vi "Ver 1.2.vi"() -> ()   [LabVIEW 2015]
uses:
  <instrlib>/Keithley 622x LV 2009/Configure/Source/Typedefs/KE622x -- Voltage Limit.ctl
  <instrlib>/Keithley 622x LV 2009/Configure/Source/Typedefs/KE622x -- Current Range.ctl
  <instrlib>/Keithley 622x LV 2009/Configure/Source/Typedefs/KE622x -- Current Ranges.ctl
  <instrlib>/Keithley 622x LV 2009/Typedefs/KE622x -- On Off Control.ctl
  <instrlib>/Keithley 622x LV 2009/Utility/Typedefs/KE622x -- Instrument Type.ctl
  <instrlib>/Keithley 622x LV 2009/Configure/Source/Typedefs/KE622x -- Current Level.ctl
  <instrlib>/Keithley 2000/Public/Configure/Configure DC Volts.vi
  <instrlib>/Keithley 2000/Keithley 2000.lvlib
  <instrlib>/Keithley 622x LV 2009/Keithley 622x.lvlib
panel:
  out "LIMIT":bool
  out "LIMIT":bool
  out "Error Code":string
  in  "Comments":string
  out "file":refnum<file>
  in  "Custom Range (0 V) 2":dbl format="%#_6p"
  in  "Auto\nRange 2":bool
  out "2000":refnum<visa-resource-name>
  out "6221":refnum<visa-resource-name>
  in  "Floating-point file recording":bool
  in  "Step  (A)":dbl=5e-05 format="%#_3p"
  in  "Stop\ncurrent (A)":dbl=0.002 format="%#_6p"
  in  "Start \ncurrent (A)":dbl=0.001 format="%#_6p"
  out "?":string
  out "?":string
  in  "Change Volt Ampers":bool
  in  "Check For SCPI Errors? (T)":bool=TRUE
  out "Interlock Tripped?":bool
  out "Compliance?":bool
  in  "Turn Off Output \nIf Compliance?":bool=TRUE
  in  "Turning ON/OFF\ncurrent output":T1=enum."On"
  out "?":cluster{dbl[], dbl[]}[](graph)
  in  "Range Selection":T2={"Auto Range?"=TRUE, "Man / Selected\nRange"=enum."2nA"}
  in  "Voltage Limit (V) 3":T4=10.0 min=0.1 max=105.0 step=0.01 format="%.2p"
  in  "Interval (s)":dbl=1.0 min=1.0
  out "?":cluster{T4[], T4[]}(graph)
  # "FILE CONFIGURATION"
  # "ADMIN PANEL"
  # "KEITHLEY 6221 CONFIGURATION (ADMIN ONLY)"
  # "I don't know what the hell it is,\njust don't touch it"
  # "START, STOP, STEP, CONFIGURATION"
  # "IF ON"
  # "Compliance = Limiting output voltage\nThis switch determines if we want to switch \noff the current output if wee exceed compliance"
  # "There is a safe switch at \nthe back of the instrument \nThis indicator shows if it is on"
  # "You have hit a damn jackpot \nby exceeding the limited voltage\nCongrats"
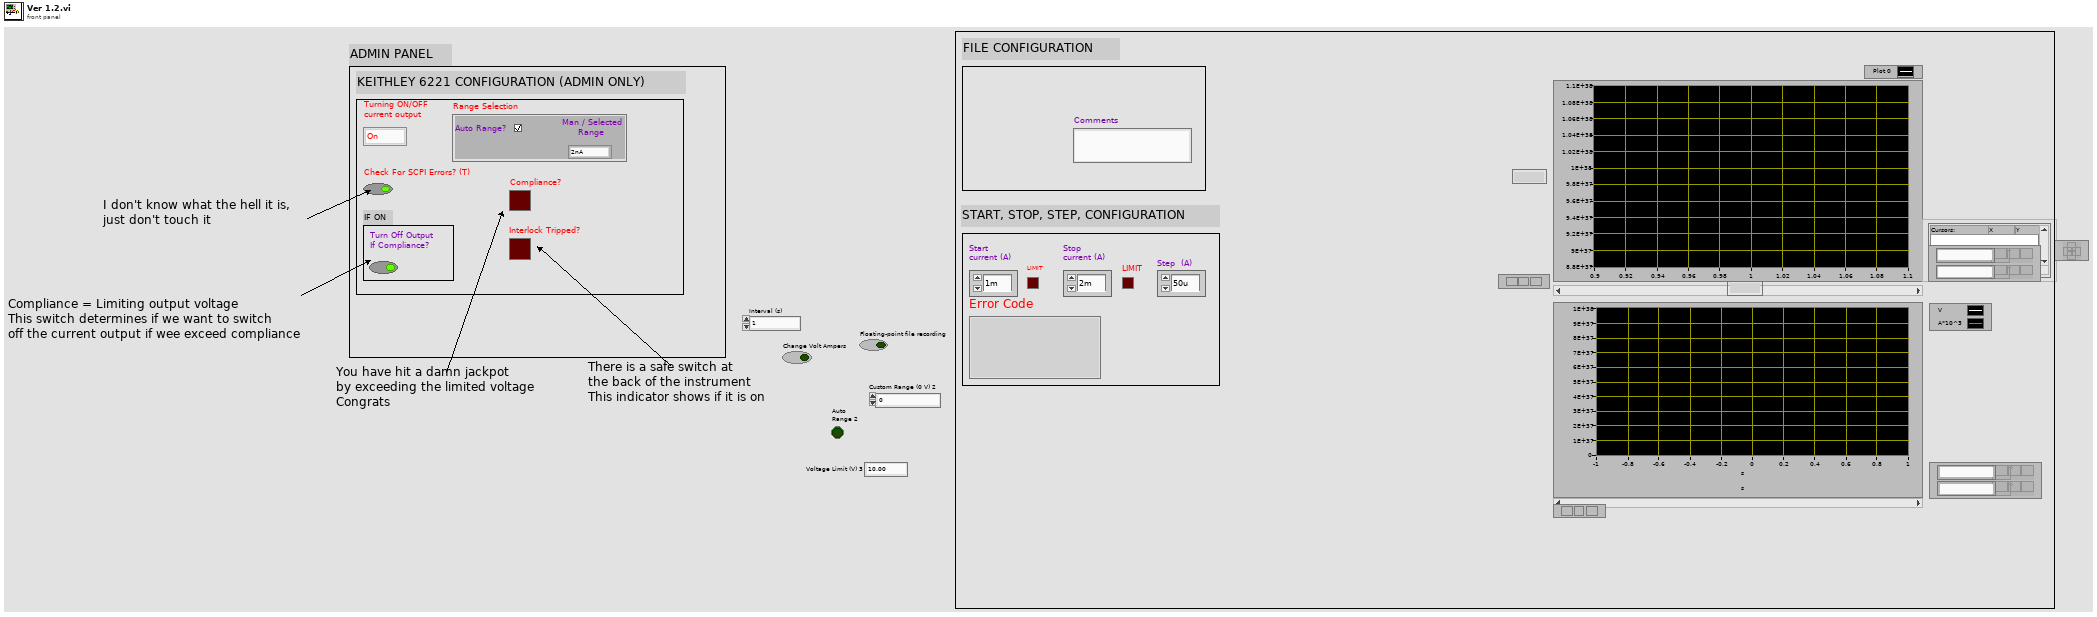
[diagram p1: front panel]
types:
  T1 = typedef "Keithley 622x.lvlib/KE622x -- On Off Control.ctl" = enum16{"Off", "On"}
  T2 = typedef "Keithley 622x.lvlib/KE622x -- Current Range.ctl" = cluster{"Auto Range?":bool, "Man / Selected\nRange":T3}
  T3 = typedef "Keithley 622x.lvlib/KE622x -- Current Ranges.ctl" = enum16{"2nA", "20nA", "200nA", "2uA", "20uA", "200uA", "2mA", "20mA", "100mA"}
  T4 = typedef "Keithley 622x.lvlib/KE622x -- Voltage Limit.ctl" = dbl
  T5 = typedef "Keithley 622x.lvlib/KE622x -- Instrument Type.ctl" = enum16{"KE6220", "KE6221"}
  T6 = typedef "Keithley 622x.lvlib/KE622x -- Current Level.ctl" = dbl
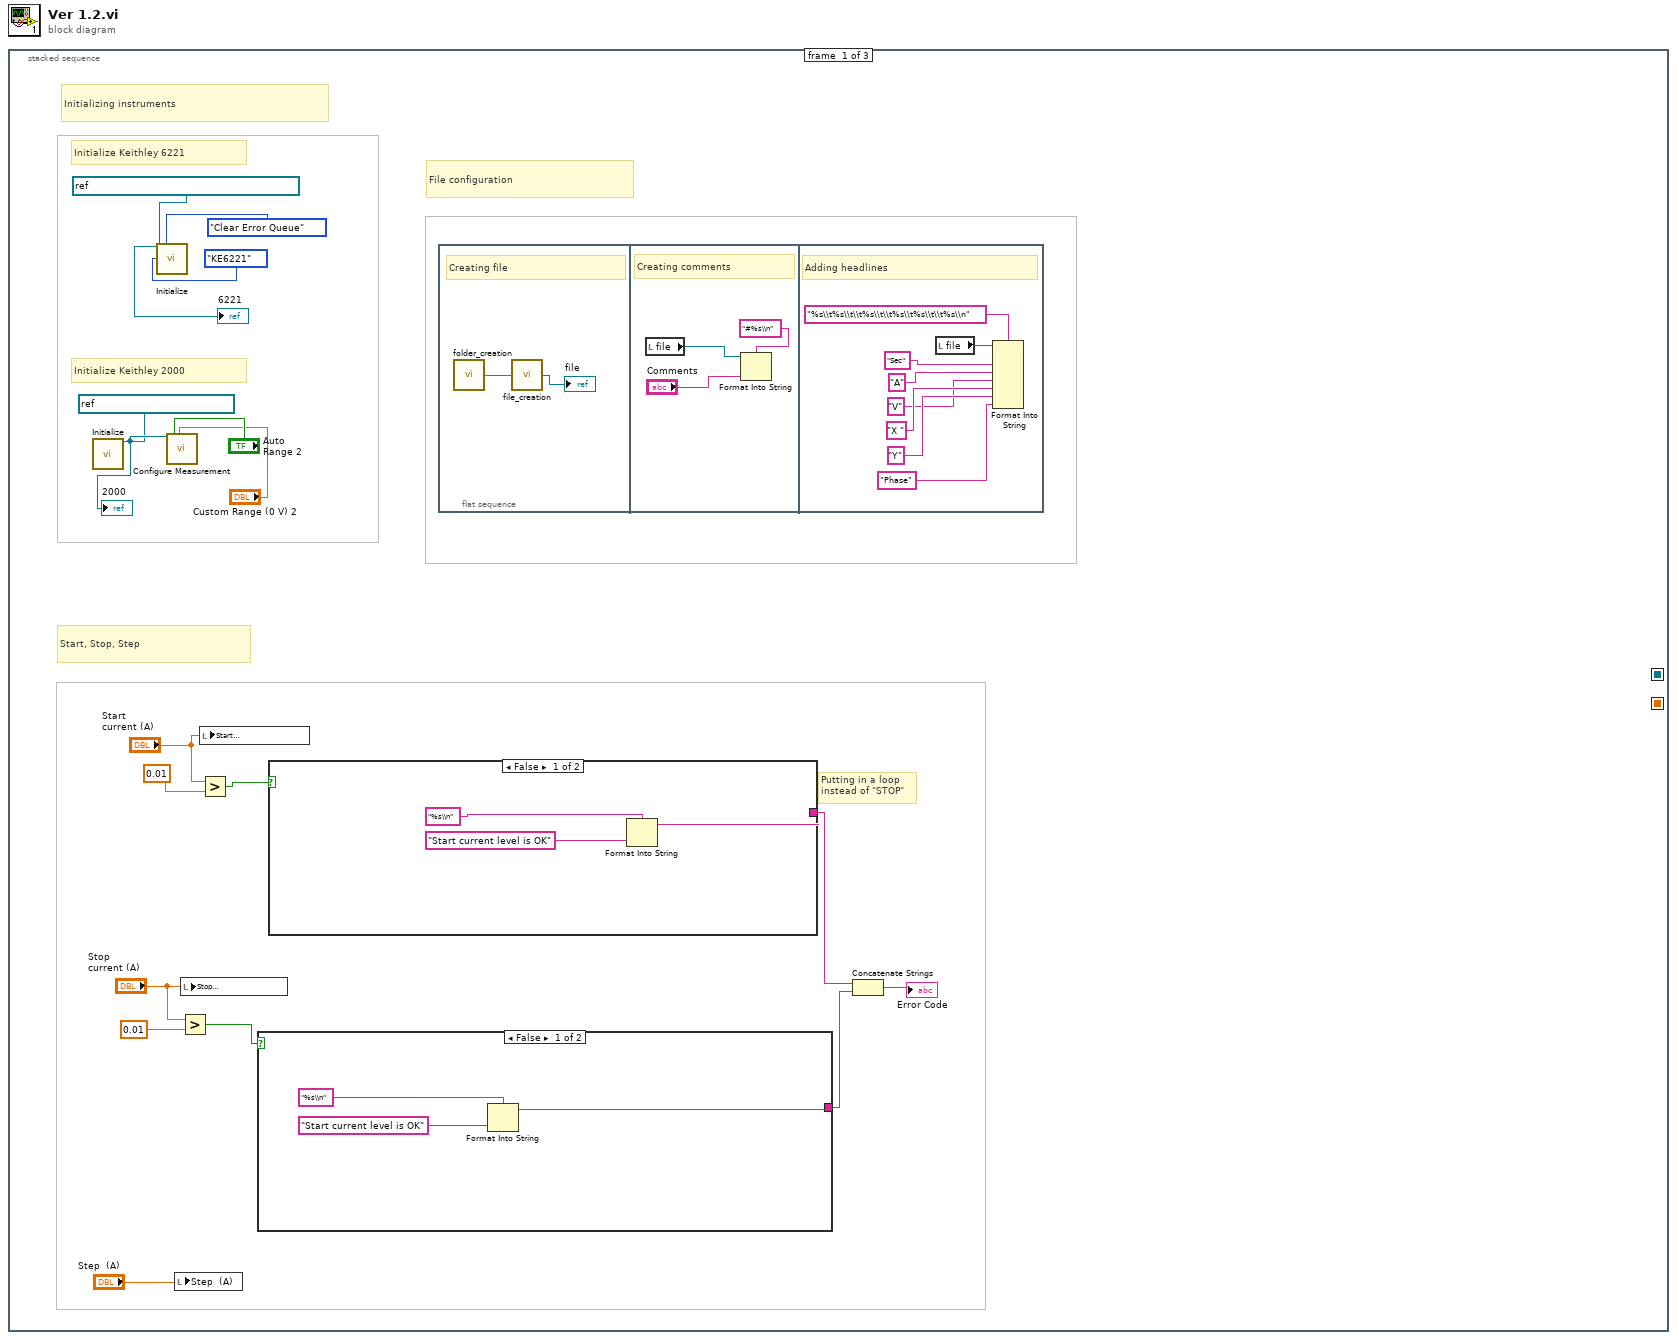
[diagram p0: block diagram]
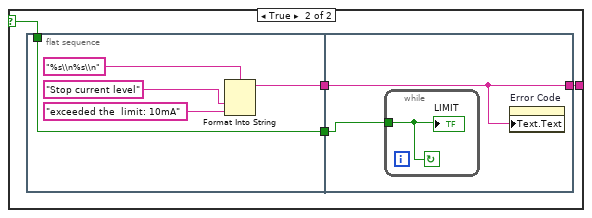
[diagram p2: hidden frame]
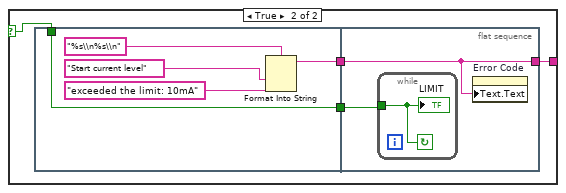
[diagram p3: hidden frame]
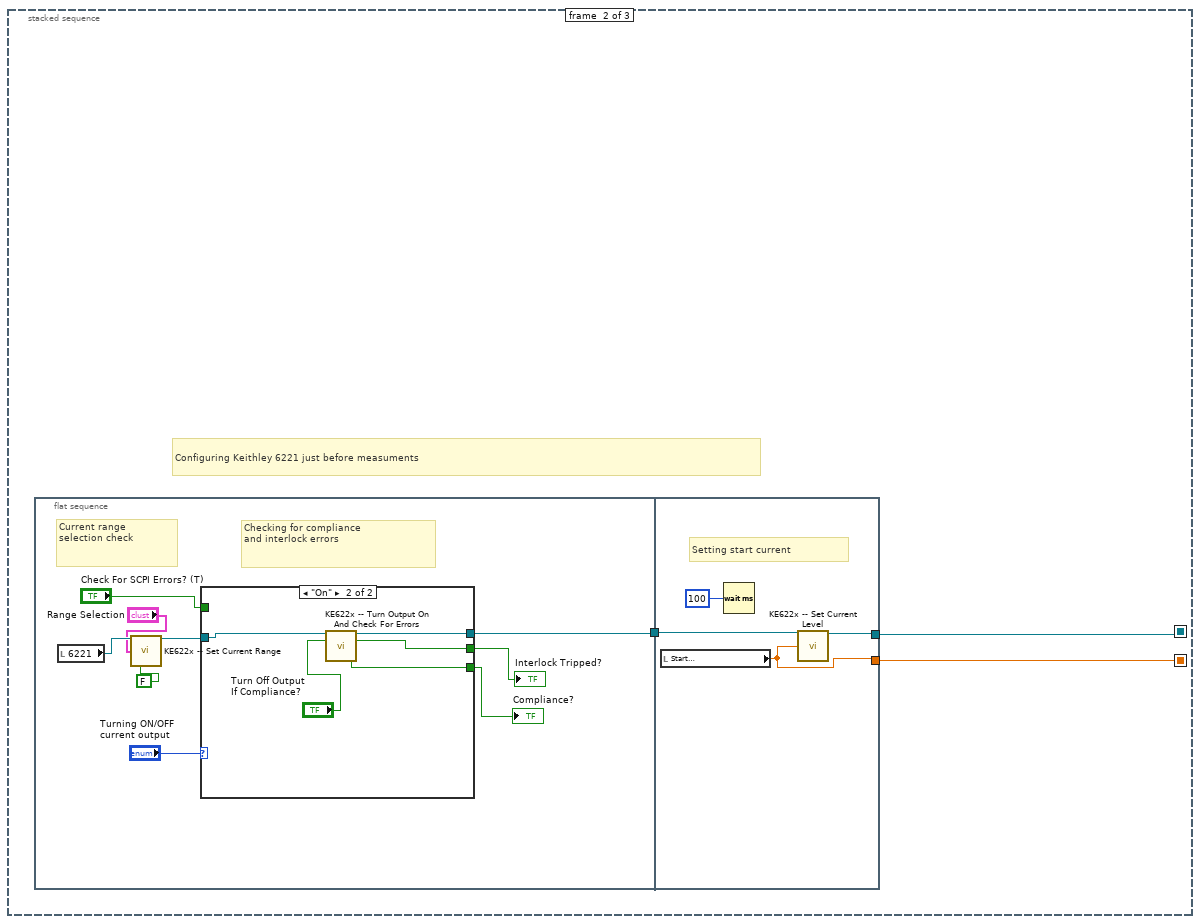
[diagram p4: hidden frame]
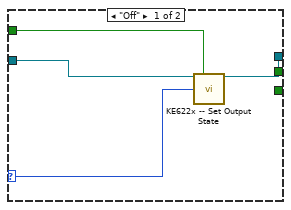
[diagram p5: hidden frame]
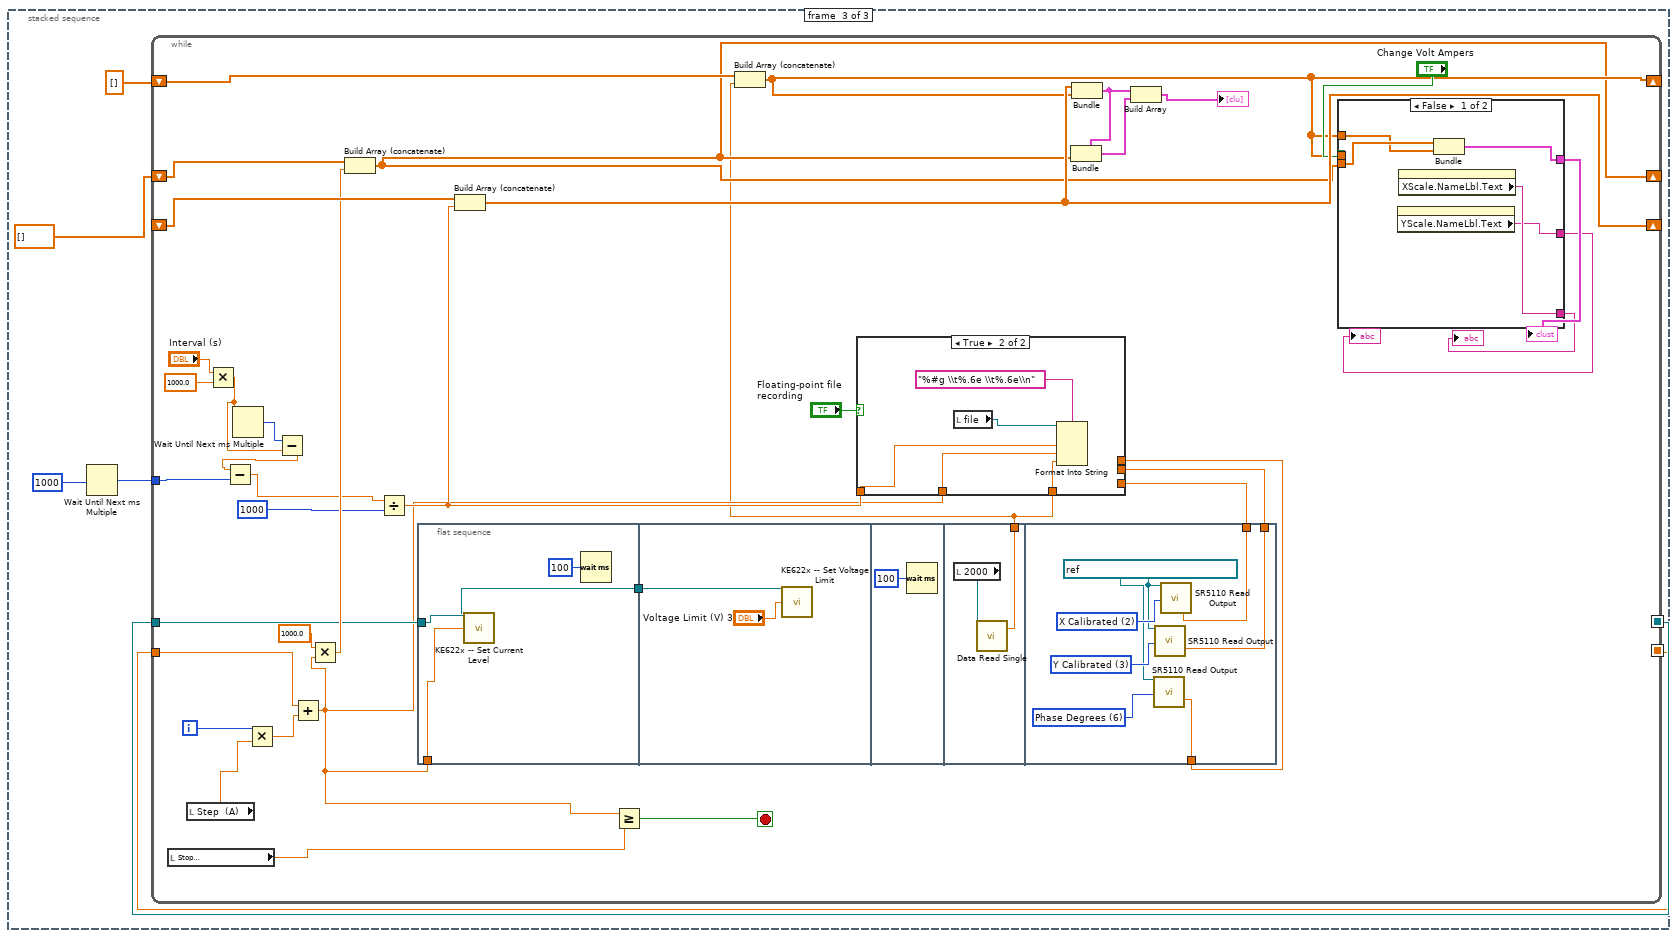
[diagram p6: hidden frame]
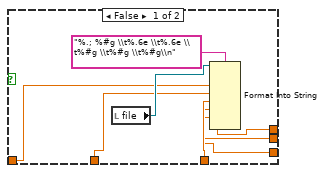
[diagram p7: hidden frame]
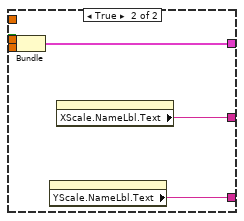
[diagram p8: hidden frame]
diagram:
  n1 = stacked-sequence {
    seq-local: [_ w64 _] -> [_ _ w87]
    seq-local: [_ w63 _] -> [_ _ w88]
    frame #0 {
      # "Putting in a loop \ninstead of \"STOP\""
      # "Start, Stop, Step"
      # "Initializing instruments"
      # "File configuration"
      # "Initialize Keithley 2000"
      # "Initialize Keithley 6221"
      n2 = call <instrlib>:"Initialize.vi"("VISA resource name"=refnum<visa-resource-name> "KEITHLEY_MULTIMETER") -> ("VISA resource name out"=w14:refnum<visa-resource-name>)  [unwired: 17 in, 1 out]
      "2000" <- w14
      n3 = call <instrlib>:"Initialize.vi"("VISA resource name"=refnum<visa-resource-name> "KEITHLEY_DC_AC_CURRENT_SOURCE", "Error Queue Option"=enum16{"Clear Error Queue", "Error Query"}."Clear Error Queue", "Instrument Type"=KE622x_--_Instrument_Type."KE6221") -> ("VISA resource name out"=→"6221":refnum<visa-resource-name>)  [unwired: 11 in, 1 out]
      n4 = call-poly <instrlib>:"Configure Measurement.vi"("VISA resource name"=w14, "Auto Range? (T: Auto)"="Auto\nRange 2", "Custom Range (0 V)"="Custom Range (0 V) 2") -> ()  [unwired: 15 in, 2 out]
      n5 = local write "Step  (A)"("Step  (A)") -> ()
      n6 = Greater?(x="Stop\ncurrent (A)", y=T4 0.01) -> (0:w4:bool)
      n7 = local write "Stop\ncurrent (A)"("Stop\ncurrent (A)") -> ()
      n8 = local write "Start \ncurrent (A)"("Start \ncurrent (A)") -> ()
      n9 = Greater?(x="Start \ncurrent (A)", y=T4 0.01) -> (0:w5:bool)
      n10 = case shown="False" w4 {
        selector: w4 -> [_ w22]
        tunnel: [w19 w25] -> w2
        frame False {
          n11 = Format Into String(format string="%s\\n", "Start current level is OK" ("false string")) -> (resulting string=w19:string)  [unwired: 2 in, 1 out]
        }
        frame True {
          n12 = flat-sequence {
            tunnel: [w27] -> w24
            tunnel: [w26] -> w23
            tunnel: w22 -> [w26]
            tunnel: [w31] -> w25
            tunnel: w24 -> [w31]
            tunnel: w23 -> [w32]
            frame #0 {
              n13 = Format Into String(format string="%s\\n%s\\n", "Stop current level" ("String"), "exceeded the  limit: 10mA" ("input 2")) -> (resulting string=w27:string)  [unwired: 2 in, 1 out]
            }
            frame #1 {
              n14 = while {
                tunnel: w32 -> [w33]
                stop <- w33 continue-if-true
                "LIMIT" <- w33
              }
              n15 = property on="Error Code" class="Str"("Text.Text"=w31) -> ()  [unwired: 2 in, 2 out]
            }
          }
        }
      }
      n16 = case shown="False" w5 {
        selector: w5 -> [_ w38]
        tunnel: [w34 w40] -> w3
        frame False {
          n17 = Format Into String(format string="%s\\n", "Start current level is OK" ("false string")) -> (resulting string=w34:string)  [unwired: 2 in, 1 out]
        }
        frame True {
          n18 = flat-sequence {
            tunnel: [w42] -> w39
            tunnel: w38 -> [w41]
            tunnel: [w41] -> w37
            tunnel: [w46] -> w40
            tunnel: w39 -> [w46]
            tunnel: w37 -> [w47]
            frame #0 {
              n19 = Format Into String(format string="%s\\n%s\\n", "Start current level" ("String"), "exceeded the limit: 10mA" ("input 2")) -> (resulting string=w42:string)  [unwired: 2 in, 1 out]
            }
            frame #1 {
              n20 = while {
                tunnel: w47 -> [w48]
                stop <- w48 continue-if-true
                "LIMIT" <- w48
              }
              n21 = property on="Error Code" class="Str"("Text.Text"=w46) -> ()  [unwired: 2 in, 2 out]
            }
          }
        }
      }
      n22 = flat-sequence {
        frame #0 {
          # "Creating file"
          n23 = call "folder_creation.vi"() -> ("String"=w50:string)
          n24 = call "file_creation.vi"("String"=w50) -> ("refnum out"=→"file":refnum<file>)
        }
        frame #1 {
          # "Creating comments"
          n25 = local read "file"() -> (w51:refnum<file>)
          n26 = Format Into String(format string="#%s\\n", initial string=w51, "Comments") -> ()  [unwired: 1 in, 2 out]
        }
        frame #2 {
          # "Adding headlines"
          n27 = local read "file"() -> (w61:refnum<file>)
          n28 = Format Into String(format string="%s\\t%s\\t\\t%s\\t\\t%s\\t%s\\t\\t%s\\n", initial string=w61, "Sec" ("input 1"), "A" ("input 2"), "V" ("input 3"), "X " ("input 3"), "Y" ("input 3"), "Phase" ("input 3")) -> ()  [unwired: 1 in, 2 out]
        }
      }
      n29 = Concatenate Strings(w3, w2) -> (→"Error Code":string)
    }
    frame #1 {
      # "Configuring Keithley 6221 just before measuments"
      n30 = flat-sequence {
        tunnel: [w65] -> w62
        tunnel: [w83] -> w64
        tunnel: [w85] -> w63
        tunnel: w62 -> [w84]
        frame #0 {
          # "Current range \nselection check"
          # "Checking for compliance\nand interlock errors"
          n31 = local read "6221"() -> (w68:refnum<visa-resource-name>)
          n32 = call <instrlib>:"KE622x -- Set Current Range.vi"("Resource In"=w68, "Current Range In"="Range Selection", "Read Back Set Values? (T)"=FALSE) -> ("Resource Out (dupl)"=w73:refnum<visa-resource-name>)  [unwired: 10 in, 2 out]
          n33 = case shown="\"On\"" "Turning ON/OFF\ncurrent output" {
            selector: "Turning ON/OFF\ncurrent output" -> [w77 _]
            tunnel: [_ w81] -> w71
            tunnel: [_ w80] -> w72
            tunnel: "Check For SCPI Errors? (T)" -> [w76 _]
            tunnel: w73 -> [w74 w79]
            tunnel: [w75 w78] -> w65
            frame "Off" {
              n34 = call <instrlib>:"KE622x -- Set Output State.vi"("Resource In"=w74, "Check For SCPI Errors? (T)"=w76, "Output State"=w77) -> ("Resource Out (dupl)"=w75:refnum<visa-resource-name>)  [unwired: 11 in, 1 out]
            }
            frame "On" {
              n35 = call <instrlib>:"KE622x -- Turn Output On And Check For Errors.vi"("Resource In"=w79, "Turn Off Output If Compliance?"="Turn Off Output \nIf Compliance?") -> ("Resource Out (dupl)"=w78:refnum<visa-resource-name>, "Interlock Tripped?"=w81:bool, "Compliance?"=w80:bool)  [unwired: 10 in, 1 out]
            }
          }
          "Interlock Tripped?" <- w71
          "Compliance?" <- w72
        }
        frame #1 {
          # "Setting start current"
          n36 = local read "Start \ncurrent (A)"() -> (w83:dbl)
          n37 = Wait (ms)(milliseconds to wait=u32 100) -> ()  [unwired: 1 out]
          n38 = call <instrlib>:"KE622x -- Set Current Level.vi"("Resource In"=w84, "Current Level (A) In"=w83) -> ("Resource Out (dupl)"=w85:refnum<visa-resource-name>)  [unwired: 12 in, 1 out]
        }
      }
    }
    frame #2 {
      n39 = Wait Until Next ms Multiple(millisecond multiple=u32 1000) -> (millisecond timer value=w89:u32)
      n40 = while {
        shift-right: [w121] -> _
        shift-left: dbl[] [] -> [w130]
        shift-right: [w126] -> _
        shift-left: _ -> [w128]
        shift-right: [w116] -> _
        shift-left: T6[] [] -> [w127]
        tunnel: w88 -> [w109]
        tunnel: w89 -> [w104]
        tunnel: w87 -> [w95]
        i -> [w118]
        stop <- w93 stop-if-true
        n41 = local read "Stop\ncurrent (A)"() -> (w94:dbl)
        n42 = local read "Step  (A)"() -> (w96:dbl)
        n43 = Multiply(x="Interval (s)", y=1000.0) -> (x*y=w105:dbl)
        n44 = Wait Until Next ms Multiple(millisecond multiple=w105) -> (millisecond timer value=w108:u32)
        n45 = Multiply(x=w118, y=w96) -> (x*y=w117:dbl)
        n46 = Subtract(x=w108, y=w105) -> (x-y=w103:dbl)
        n47 = Subtract(x=w103, y=w104) -> (x-y=w102:dbl)
        n48 = Add(x=w95, y=w117) -> (x+y=w106:dbl)
        n49 = Multiply(x=T4 1000.0, y=w106) -> (x*y=w115:T4)
        n50 = Build Array (concatenate)(w127, w115) -> (w116:T4[])
        n51 = Divide(x=w102, y=1000) -> (x/y=w112:dbl)
        n52 = flat-sequence {
          tunnel: w106 -> [w147]
          tunnel: w109 -> [w146]
          tunnel: [w145] -> w107
          tunnel: w107 -> [w148]
          tunnel: [w151] -> w99
          tunnel: [w159] -> w100
          tunnel: [w154] -> w98
          tunnel: [w153] -> w97
          frame #0 {
            n53 = call <instrlib>:"KE622x -- Set Current Level.vi"("Resource In"=w146, "Current Level (A) In"=w147) -> ("Resource Out (dupl)"=w145:refnum<visa-resource-name>)  [unwired: 12 in, 1 out]
            n54 = Wait (ms)(milliseconds to wait=u32 100) -> ()  [unwired: 1 out]
          }
          frame #1 {
            n55 = call <instrlib>:"KE622x -- Set Voltage Limit.vi"("Resource In"=w148, "Voltage Limit (V)"="Voltage Limit (V) 3") -> ()  [unwired: 12 in, 2 out]
          }
          frame #2 {
            n56 = Wait (ms)(milliseconds to wait=u32 100) -> ()  [unwired: 1 out]
          }
          frame #3 {
            n57 = local read "2000"() -> (w152:refnum<visa-resource-name>)
            n58 = call <instrlib>:"Data Read Single.vi"("VISA resource name"=w152) -> ("Measurement"=w151:dbl)  [unwired: 14 in, 4 out]
          }
          frame #4 {
            w156 = u16 6 items=["X %", "Y %", "X Calibrated", "Y Calibrated", "Mag %", "Mag Calibrated", "Phase Degrees", "Ratio", "ADC 1", "ADC 2", "ADC 3", "ADC 4 ", "Noise %", "Noise Calibrated", "Ref Frequency", "", ""] ("Display Type")
            w157 = u16 3 items=["X %", "Y %", "X Calibrated", "Y Calibrated", "Mag %", "Mag Calibrated", "Phase Degrees", "Ratio", "ADC 1", "ADC 2", "ADC 3", "ADC 4 ", "Noise %", "Noise Calibrated", "Ref Frequency", "", ""] ("Display Type")
            w158 = u16 2 items=["X %", "Y %", "X Calibrated", "Y Calibrated", "Mag %", "Mag Calibrated", "Phase Degrees", "Ratio", "ADC 1", "ADC 2", "ADC 3", "ADC 4 ", "Noise %", "Noise Calibrated", "Ref Frequency", "", ""] ("Display Type")
            w155 = refnum<visa-resource-name> "LOCK_IN_5110_PRINCETON" ("VISA session (for class)")
            n59 = call "SR5110 Read Output"("VISA session (for class)"=w155, "Display Type"=w156) -> ("Output (FP)"=w153:dbl)  [unwired: 9 in, 8 out]
            n60 = call "SR5110 Read Output"("VISA session (for class)"=w155, "Display Type"=w157) -> ("Output (FP)"=w154:dbl)  [unwired: 9 in, 8 out]
            n61 = call "SR5110 Read Output"("VISA session (for class)"=w155, "Display Type"=w158) -> ("Display"=w159:dbl)  [unwired: 9 in, 8 out]
          }
        }
        n62 = Build Array (concatenate)(w128, w112) -> (w126:dbl[])
        n63 = Greater Or Equal?(x=w106, y=w94) -> (x >= y?=w93:bool)
        n64 = Build Array (concatenate)(w130, w99) -> (w121:dbl[])
        n65 = case shown="True" "Floating-point file recording" {
          tunnel: w112 -> [w134 w141]
          tunnel: w99 -> [w136 w140]
          tunnel: w106 -> [w135 w139]
          tunnel: w100 -> [w133 _]
          tunnel: w98 -> [w132 _]
          tunnel: w97 -> [w131 _]
          frame False {
            n66 = local read "file"() -> (w137:refnum<file>)
            n67 = Format Into String(format string="%.; %#g \\t%.6e \\t%.6e \\t%#g \\t%#g \\t%#g\\n", initial string=w137, w134, w135, w136, w133, w132, w131) -> ()  [unwired: 1 in, 2 out]
          }
          frame True {
            n68 = local read "file"() -> (w142:refnum<file>)
            n69 = Format Into String(format string="%#g \\t%.6e \\t%.6e\\n", initial string=w142, w141, w139, w140) -> ()  [unwired: 1 in, 2 out]
          }
        }
        n70 = Bundle(w126, w121) -> (w124:cluster{dbl[], dbl[]})  [unwired: 1 in]
        n71 = Bundle(cluster=w124, w116) -> (w125:cluster{dbl[], dbl[]})  [unwired: 1 in]
        n72 = Build Array(w124, w125) -> (→"?":cluster{dbl[], dbl[]}[])
        n73 = case shown="False" "Change Volt Ampers" {
          tunnel: [w164 w169] -> w129
          tunnel: w121 -> [_ w168]
          tunnel: w116 -> [w163 w167]
          tunnel: w121 -> [w162 _]
          tunnel: [w160 w166] -> w120
          tunnel: [w161 w165] -> w119
          frame False {
            n74 = property class="XYGraph (strict)"() -> ("YScale.NameLbl.Text"=w160:string)  [unwired: 2 in, 2 out]
            n75 = property class="XYGraph (strict)"() -> ("XScale.NameLbl.Text"=w161:string)  [unwired: 2 in, 2 out]
            n76 = Bundle(w163, w162) -> (w164:cluster{T4[], dbl[]})  [unwired: 1 in]
          }
          frame True {
            n77 = Bundle(w168, w167) -> (w169:cluster{dbl[], T4[]})  [unwired: 1 in]
            n78 = property class="XYGraph (strict)"() -> ("YScale.NameLbl.Text"=w165:string)  [unwired: 2 in, 2 out]
            n79 = property class="XYGraph (strict)"() -> ("XScale.NameLbl.Text"=w166:string)  [unwired: 2 in, 2 out]
          }
        }
        "?" <- w129
        "?" <- w120
        "?" <- w119
      }
    }
  }
